vi "Web receiver.vi"(11 "queue in":refnum<queue>) -> (2 "Connected?":bool, 3 "Device trying to connect":bool)   [LabVIEW 2014]
uses:
  controls/UI Data.ctl
  controls/Web command parser enum.ctl
  controls/UI DataSam.ctl
  controls/Variables to check enum.ctl
  globals/RT Network Stream Endpoints.vi
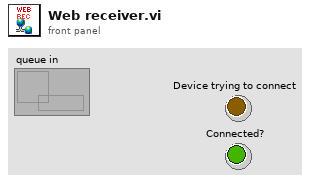
[diagram p1: front panel]
types:
  T1 = typedef "Variables to check enum.ctl" = enum16{"Control", "Direction"}
  T2 = typedef "UI DataSam.ctl" = cluster{"Message":string, "Data":variant}
  T3 = typedef "Web command parser enum.ctl" = enum16{"Wait for connect", "Write Commands"}
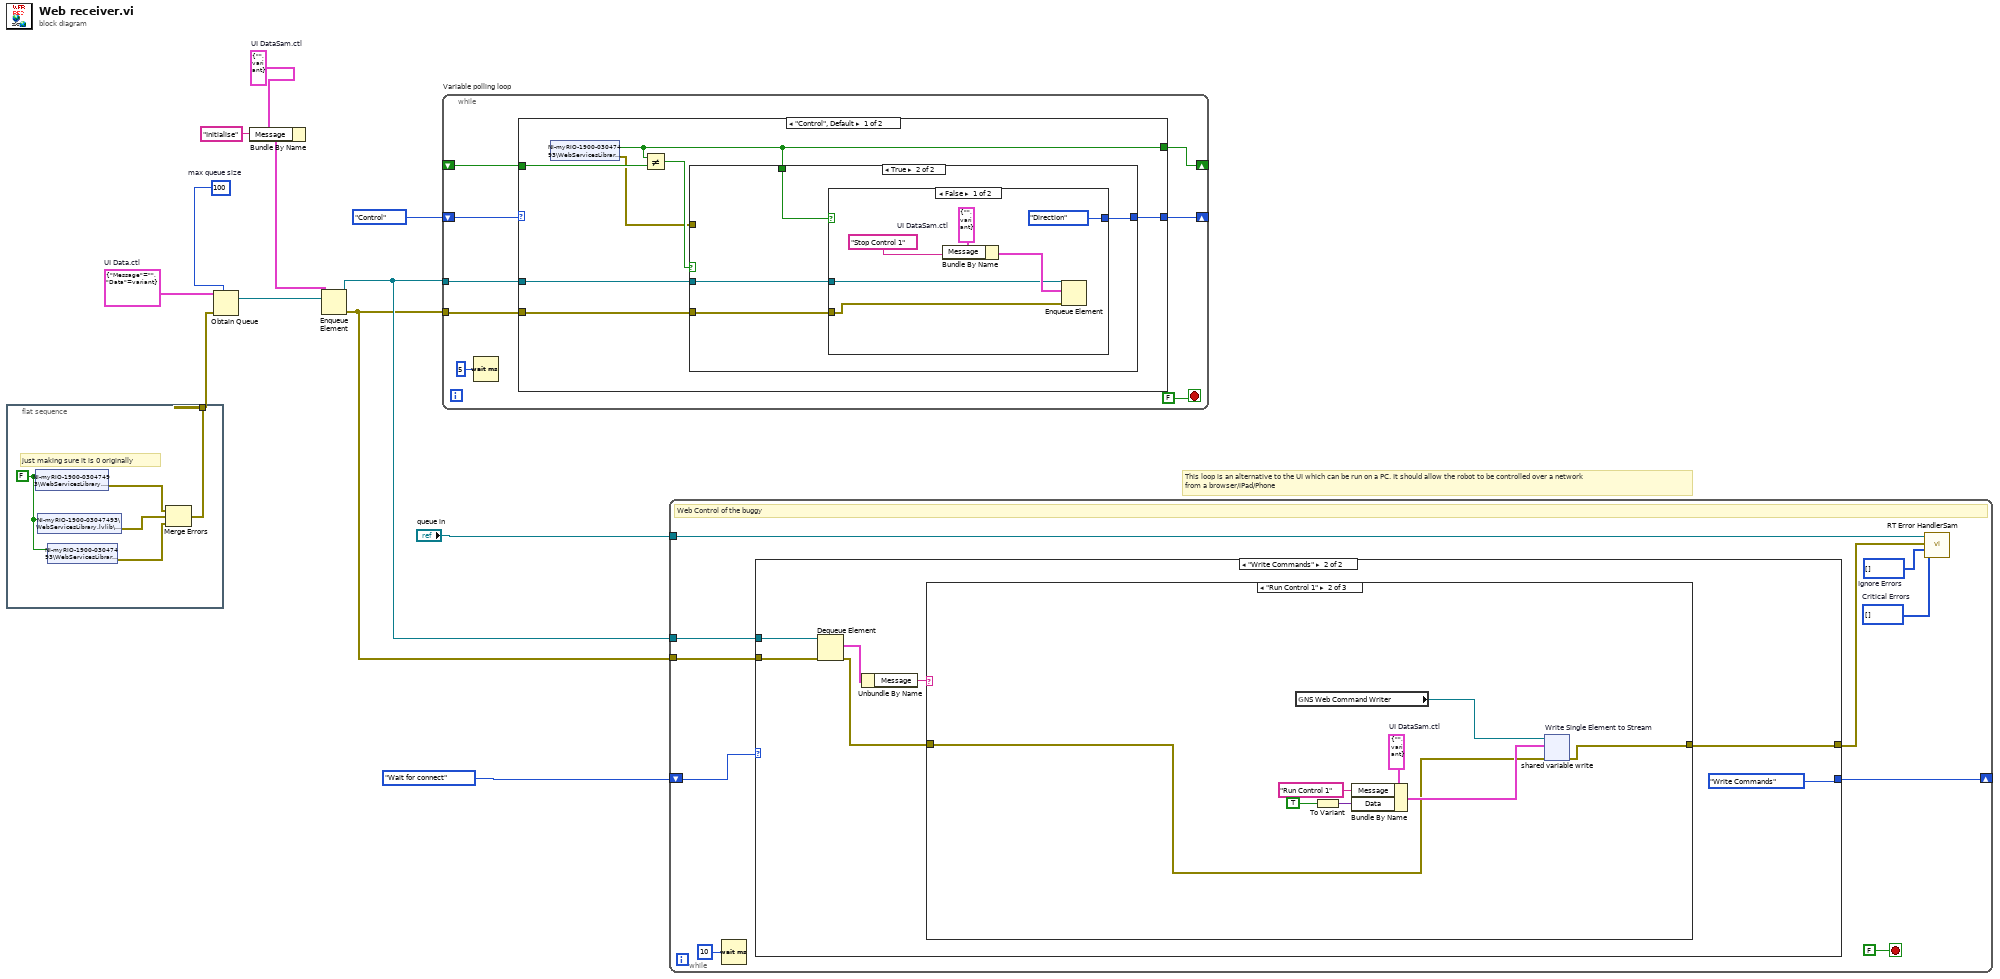
[diagram p0: block diagram]
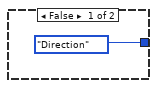
[diagram p2: hidden frame]
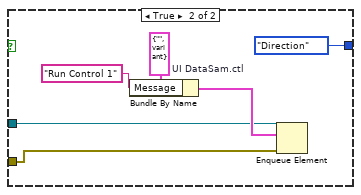
[diagram p3: hidden frame]
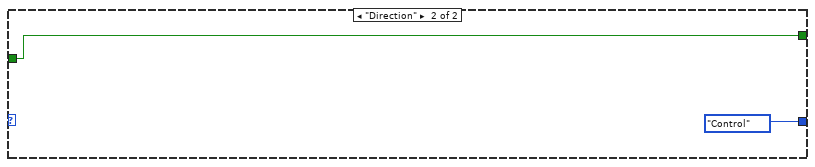
[diagram p4: hidden frame]
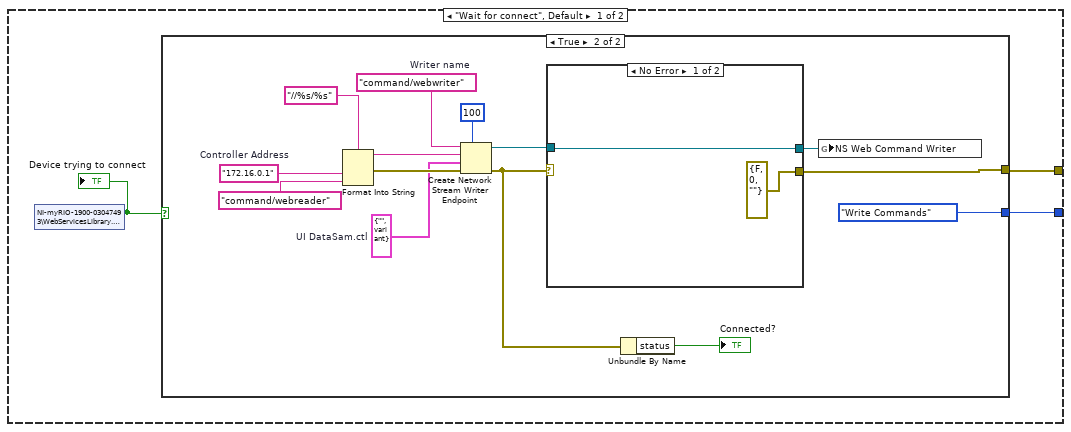
[diagram p5: hidden frame]
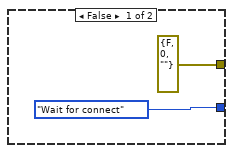
[diagram p6: hidden frame]
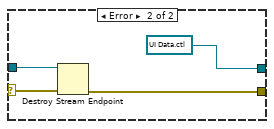
[diagram p7: hidden frame]
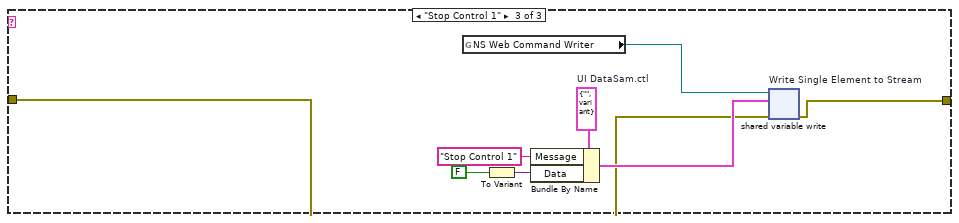
[diagram p9: hidden frame]
diagram:
  w11 = T2 {"Message"="", "Data"=variant}  # UI DataSam.ctl
  w9 = T2 {"Message"="", "Data"=variant}  # UI Data.ctl
  w6 = 100  # max queue size
  # "This loop is an alternative to the UI which can be run on a PC. It should allow the robot to be controlled over a network\nfrom a browser/iPad/Phone"
  n1 = flat-sequence {
    tunnel: [w13] -> w10
    frame #0 {
      w16 = FALSE ("Connect")
      # "just making sure it is 0 originally"
      n2 = shared-variable "NI-myRIO-1900-03047493\\WebServicesLibrary.lvlib\\Connect"(w16) -> (error out=w14:errorcluster)  [unwired: 1 in]
      n3 = shared-variable "NI-myRIO-1900-03047493\\WebServicesLibrary.lvlib\\Connected"(w16) -> (error out=w15:errorcluster)  [unwired: 1 in]
      n4 = shared-variable "NI-myRIO-1900-03047493\\WebServicesLibrary.lvlib\\Control"(w16) -> (error out=w17:errorcluster)  [unwired: 1 in]
      n5 = Merge Errors(w14, w15, w17) -> (w13:errorcluster)
    }
  }
  n6 = Obtain Queue(max queue size (-1, unlimited)=w6, element data type=w9, error in (no error)=w10) -> (queue out=w5:refnum<queue>)  [unwired: 2 in, 2 out]
  n7 = Bundle By Name(cluster=w11, "Message"="Initialise") -> (w8:T2)
  n8 = Enqueue Element(queue=w5, element=w8) -> (queue out=w3:refnum<queue>, error out=w2:errorcluster)  [unwired: 2 in, 1 out]
  n9 = while "Variable polling loop" {
    tunnel: w3 -> [w25]
    tunnel: w2 -> [w24]
    shift-right: [w20] -> _
    shift-left: Variables_to_check_enum."Control" ("Command Parser Enum") -> [w23]
    shift-right: [w21] -> _
    shift-left: _ -> [w22]
    stop <- FALSE stop-if-true
    n10 = Wait (ms)(milliseconds to wait=u32 5) -> ()  [unwired: 1 out]
    n11 = case shown="\"Control\", Default" w23 {
      tunnel: w25 -> [w29 _]
      tunnel: w24 -> [w28 _]
      tunnel: w22 -> [w31 w50]
      tunnel: [w26 w50] -> w21
      tunnel: [w27 Variables_to_check_enum."Control" ("Command Parser Enum")] -> w20
      frame "Control", Default {
        n12 = shared-variable "NI-myRIO-1900-03047493\\WebServicesLibrary.lvlib\\Control"() -> (w26:bool, error out=w30:errorcluster)  [unwired: 1 in]
        n13 = Not Equal?(x=w26, y=w31) -> (x != y?=w32:bool)
        n14 = case shown="True" w32 {
          tunnel: w30 -> [_ _]
          tunnel: w29 -> [_ w37]
          tunnel: w28 -> [_ w36]
          tunnel: [Variables_to_check_enum."Direction" ("Command Parser Enum") w35] -> w27
          tunnel: w26 -> [_ w34]
          frame False {
          }
          frame True {
            n15 = case shown="False" w34 {
              tunnel: w37 -> [w40 w46]
              tunnel: w36 -> [w39 w45]
              tunnel: [Variables_to_check_enum."Direction" ("Command Parser Enum") Variables_to_check_enum."Direction" ("Command Parser Enum")] -> w35
              frame False {
                w41 = T2 {"Message"="", "Data"=variant}  # UI DataSam.ctl
                n16 = Bundle By Name(cluster=w41, "Message"="Stop Control 1") -> (w42:T2)
                n17 = Enqueue Element(queue=w40, element=w42, error in (no error)=w39) -> ()  [unwired: 1 in, 3 out]
              }
              frame True {
                w47 = T2 {"Message"="", "Data"=variant}  # UI DataSam.ctl
                n18 = Bundle By Name(cluster=w47, "Message"="Run Control 1") -> (w48:T2)
                n19 = Enqueue Element(queue=w46, element=w48, error in (no error)=w45) -> ()  [unwired: 1 in, 3 out]
              }
            }
          }
        }
      }
      frame "Direction" {
      }
    }
  }
  n20 = while {
    tunnel: "queue in" -> [w58]
    shift-right: [w55] -> _
    shift-left: Web_command_parser_enum."Wait for connect" ("Command Parser Enum") -> [w54]
    tunnel: w3 -> [w53]
    tunnel: w2 -> [w52]
    stop <- FALSE stop-if-true
    w59 = i32[] []  # Ignore Errors
    w60 = i32[] []  # Critical Errors
    # "Web Control of the buggy"
    n21 = Wait (ms)(milliseconds to wait=u32 10) -> ()  [unwired: 1 out]
    n22 = case shown="\"Write Commands\"" w54 {
      tunnel: [w64 w87] -> w57
      tunnel: [w62 Web_command_parser_enum."Write Commands" ("Command Parser Enum")] -> w55
      tunnel: w53 -> [_ w92]
      tunnel: w52 -> [_ w91]
      frame "Wait for connect", Default {
        n23 = shared-variable "NI-myRIO-1900-03047493\\WebServicesLibrary.lvlib\\Connect"() -> (w63:bool)  [unwired: 1 in, 1 out]
        "Device trying to connect" <- w63
        n24 = case shown="True" w63 {
          tunnel: [errorcluster {"status"=FALSE, "code"=0, "source"=""} ("error out") w71] -> w64
          tunnel: [Web_command_parser_enum."Wait for connect" ("Command Parser Enum") Web_command_parser_enum."Write Commands" ("Command Parser Enum")] -> w62
          frame False {
          }
          frame True {
            w70 = "172.16.0.1"  # Controller Address
            w74 = T2 {"Message"="", "Data"=variant}  # UI DataSam.ctl
            w75 = "command/webwriter"  # Writer name
            n25 = Format Into String(format string="//%s/%s", w70, "command/webreader" ("input 2")) -> (resulting string=w77:string, error out=w78:errorcluster)  [unwired: 2 in]
            n26 = Create Network Stream Writer Endpoint(7:100 ("writer buffer size"), 8:w78, 9:w74, 10:w77, 11:w75) -> (0:w72:errorcluster, 3:w73:refnum<k21>)  [unwired: 2 in]
            n27 = case shown="No Error" w72 {
              selector: w72 -> [_ w86]
              tunnel: w73 -> [w82 w85]
              tunnel: [w82 refnum<k21> refnum ("Writer name")] -> w67
              tunnel: [errorcluster {"status"=FALSE, "code"=0, "source"=""} ("error out") w83] -> w71
              frame No Error {
              }
              frame Error {
                n28 = Destroy Stream Endpoint(8:w86, 11:w85) -> (0:w83:errorcluster)
              }
            }
            n29 = Unbundle By Name(w72) -> ("status"=→"Connected?":bool)
            n30 = global write "RT Network Stream Endpoints.vi" "NS Web Command Writer"(w67) -> ()
          }
        }
      }
      frame "Write Commands" {
        n31 = Dequeue Element(queue=w92, error in (no error)=w91) -> (element=w90:T2, error out=w88:errorcluster)  [unwired: 1 in, 2 out]
        n32 = Unbundle By Name(w90) -> ("Message"=w89:string)
        n33 = case shown="\"Run Control 1\"" w89 {
          tunnel: w88 -> [w94 w95 w103]
          tunnel: [w94 w96 w104] -> w87
          frame "", Default {
          }
          frame "Run Control 1" {
            w100 = T2 {"Message"="", "Data"=variant}  # UI DataSam.ctl
            n34 = global read "RT Network Stream Endpoints.vi" "NS Web Command Writer"() -> (w102:refnum<k21>)
            n35 = To Variant(anything=TRUE) -> (Variant=w99:variant)
            n36 = Bundle By Name(cluster=w100, "Message"="Run Control 1", "Data"=w99) -> (w101:T2)
            n37 = shared-variable-write "Write Single Element to Stream"(w102, w95, w101) -> (w96:errorcluster)  [unwired: 1 in, 2 out]
          }
          frame "Stop Control 1" {
            w108 = T2 {"Message"="", "Data"=variant}  # UI DataSam.ctl
            n38 = global read "RT Network Stream Endpoints.vi" "NS Web Command Writer"() -> (w110:refnum<k21>)
            n39 = To Variant(anything=FALSE) -> (Variant=w107:variant)
            n40 = Bundle By Name(cluster=w108, "Message"="Stop Control 1", "Data"=w107) -> (w109:T2)
            n41 = shared-variable-write "Write Single Element to Stream"(w110, w103, w109) -> (w104:errorcluster)  [unwired: 1 in, 2 out]
          }
        }
      }
    }
    n42 = call "RT Error HandlerSam.vi"("Ignore Errors"=w59, "Critical Errors"=w60, "error to process"=w57, "queue in"=w58) -> ()  [unwired: 7 in, 1 out]
  }
